vi "快速排序法-带索引映射.vi"(6 "模式":enum16{"从小到大", "从大到小"}(ring), 11 "数组":dbl[](array[numeric])=[1.0, 2.0, 3.0, 4.0, 5.0, 5.0, 5.0, 5.0, 1.0, 3.0, 7.0, 9.0, 12.0]) -> (0 "输出簇":errorcluster, 2 "索引映射":i32[](array[numeric]), 3 "排序后":dbl[](array[numeric]))   [LabVIEW 2013]
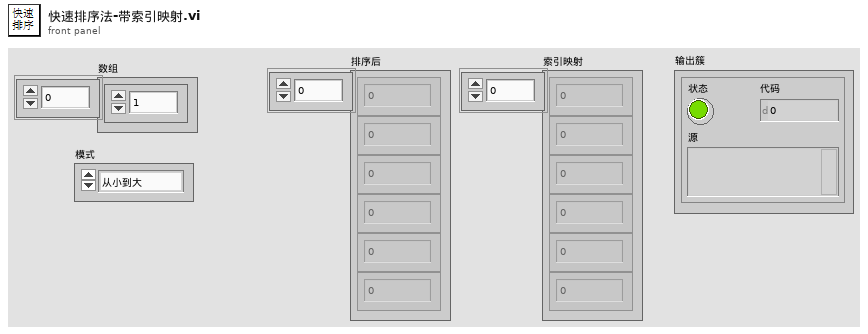
[diagram p1: front panel]
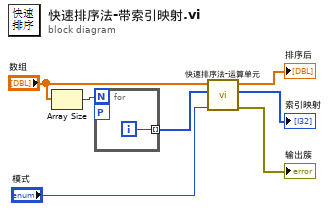
[diagram p0: block diagram]
diagram:
  n1 = Array Size(array="数组") -> (size(s)=w6:i32)
  n2 = for {
    N: w6 -> [_]
    workers-P: _ -> [_]
    tunnel: [w8] -> w5 mode=indexing
    i -> [w8]
  }
  n3 = call "快速排序法-运算单元.vi"("模式"="模式", "数组跟随索引"=w5, "数组"="数组") -> ("输出簇"=→"输出簇":errorcluster, "索引映射"=→"索引映射":i32[], "排序后"=→"排序后":dbl[])  [unwired: 6 in]
